vi "Configure Serial Bus (SPI - Source).vi"(0 "VISA resource name":refnum<visa-resource-name>, 1 "MISO Source Channel (0: Channel 1)":i32(ring) items=["Channel 1"=0, "Channel 2"=1, "Channel 3"=2, "Channel 4"=3, "D0"=13, "D1"=14, "D2"=15, "D3"=16, "D4"=17, "D5"=18, "D6"=19, "D7"=20, "D8"=21, "D9"=22, "D10"=23, "D11"=24, "D12"=25, "D13"=26, "D14"=27, "D15"=28, "External"=29], 2 "MOSI Source Channel (1: Channel 2)":i32(ring)=1 items=["Channel 1"=0, "Channel 2"=1, "Channel 3"=2, "Channel 4"=3, "D0"=13, "D1"=14, "D2"=15, "D3"=16, "D4"=17, "D5"=18, "D6"=19, "D7"=20, "D8"=21, "D9"=22, "D10"=23, "D11"=24, "D12"=25, "D13"=26, "D14"=27, "D15"=28, "External"=29], 3 "Clock Source Channel (2: Channel 3)":i32(ring)=2 items=["Channel 1"=0, "Channel 2"=1, "Channel 3"=2, "Channel 4"=3, "D0"=13, "D1"=14, "D2"=15, "D3"=16, "D4"=17, "D5"=18, "D6"=19, "D7"=20, "D8"=21, "D9"=22, "D10"=23, "D11"=24, "D12"=25, "D13"=26, "D14"=27, "D15"=28, "External"=29], 5 "Serial Bus Name (1: Serial Bus 1)":i32(ring)=1 items=["Serial Bus 1"=1, "Serial Bus 2"=2], 7 "Enable Frame Source (F: Disable)":bool, 9 "Frame Source Channel (3: Channel 4)":i32(ring)=3 items=["Channel 1"=0, "Channel 2"=1, "Channel 3"=2, "Channel 4"=3, "D0"=13, "D1"=14, "D2"=15, "D3"=16, "D4"=17, "D5"=18, "D6"=19, "D7"=20, "D8"=21, "D9"=22, "D10"=23, "D11"=24, "D12"=25, "D13"=26, "D14"=27, "D15"=28, "External"=29], 11 "error in (no error)":errorcluster, 12 "DATA Source Channel (1: Channel 1)":i32(ring)=1 items=["Channel 1"=0, "Channel 2"=1, "Channel 3"=2, "Channel 4"=3, "D0"=13, "D1"=14, "D2"=15, "D3"=16, "D4"=17, "D5"=18, "D6"=19, "D7"=20, "D8"=21, "D9"=22, "D10"=23, "D11"=24, "D12"=25, "D13"=26, "D14"=27, "D15"=28, "External"=29]) -> (4 "VISA resource name out":refnum<visa-resource-name>, 15 "error out":errorcluster)   [LabVIEW 2015, in "Agilent 2000 3000 X-Series.lvlib"]
doc: "Configures the source settings of SPI bus."
uses:
  Agilent 2000 3000 X-Series.lvlib
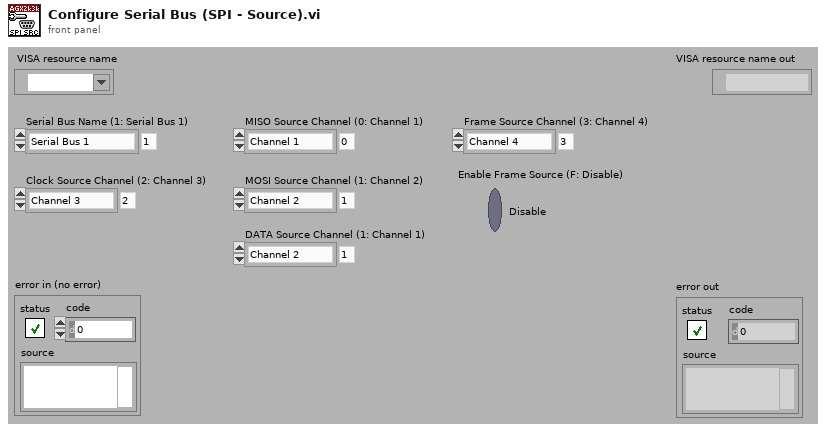
[diagram p1: front panel]
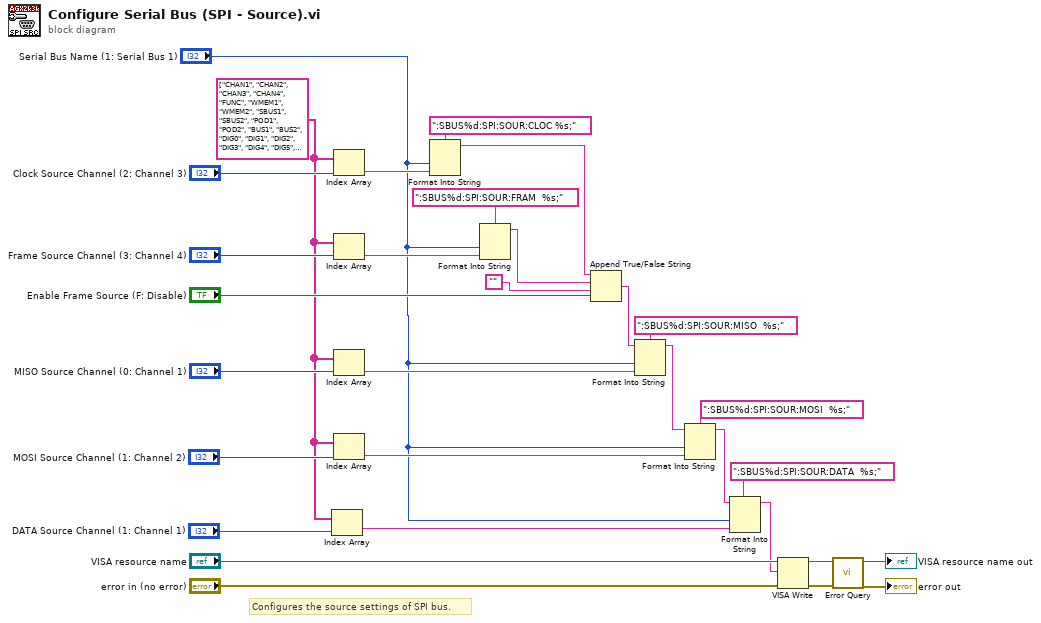
[diagram p0: block diagram]
diagram:
  w5 = string[] ["CHAN1", "CHAN2", "CHAN3", "CHAN4", "FUNC", "WMEM1", "WMEM2", "SBUS1", "SBUS2", "POD1", "POD2", "BUS1", "BUS2", "DIG0", "DIG1", "DIG2", "DIG3", "DIG4", "DIG5", "DIG6", "DIG7", "DIG8", "DIG9", "DIG10", "DIG11", "DIG12", "DIG13", "DIG14", "DIG15", "EXT", "LINE", "WGEN"]
  # "Configures the source settings of SPI bus."
  n1 = Index Array(array=w5, index="DATA Source Channel (1: Channel 1)") -> (element=w6:string)
  n2 = Index Array(array=w5, index="Clock Source Channel (2: Channel 3)") -> (element=w15:string)
  n3 = Index Array(array=w5, index="Frame Source Channel (3: Channel 4)") -> (element=w8:string)
  n4 = Index Array(array=w5, index="MISO Source Channel (0: Channel 1)") -> (element=w11:string)
  n5 = Index Array(array=w5, index="MOSI Source Channel (1: Channel 2)") -> (element=w13:string)
  n6 = Format Into String(format string=":SBUS%d:SPI:SOUR:CLOC %s;", "Serial Bus Name (1: Serial Bus 1)", w15) -> (resulting string=w20:string)  [unwired: 2 in, 1 out]
  n7 = Format Into String(format string=":SBUS%d:SPI:SOUR:FRAM  %s;", "Serial Bus Name (1: Serial Bus 1)", w8) -> (resulting string=w19:string)  [unwired: 2 in, 1 out]
  n8 = Append True/False String(1:"Enable Frame Source (F: Disable)", 2:"", 3:w19, 4:w20) -> (0:w17:string)
  n9 = Format Into String(format string=":SBUS%d:SPI:SOUR:MISO  %s;", initial string=w17, "Serial Bus Name (1: Serial Bus 1)", w11) -> (resulting string=w28:string)  [unwired: 1 in, 1 out]
  n10 = Format Into String(format string=":SBUS%d:SPI:SOUR:MOSI  %s;", initial string=w28, "Serial Bus Name (1: Serial Bus 1)", w13) -> (resulting string=w3:string)  [unwired: 1 in, 1 out]
  n11 = Format Into String(format string=":SBUS%d:SPI:SOUR:DATA  %s;", initial string=w3, "Serial Bus Name (1: Serial Bus 1)", w6) -> (resulting string=w4:string)  [unwired: 1 in, 1 out]
  n12 = VISA Write(VISA resource name="VISA resource name", write buffer=w4, error in (no error)="error in (no error)") -> (VISA resource name out=w24:refnum<visa-resource-name>, error out=w23:errorcluster)  [unwired: 1 out]
  n13 = call "Error Query.vi"("error in (no error)"=w23, "VISA resource name"=w24) -> ("error out"=→"error out":errorcluster, "VISA resource name out"=→"VISA resource name out":refnum<visa-resource-name>)  [unwired: 8 out]
